vi "Save Timestamps to TXT.vi"(10 "Path To Exp":path, 11 "Timestamps (ms)":u64[](array[numeric])) -> (2 "Path To Exp out":path)   [LabVIEW 2020]
uses:
  <vilib>/Utility/file.llb/Write Delimited Spreadsheet (I64).vi
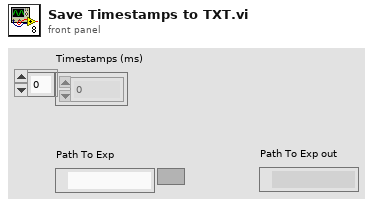
[diagram p1: front panel]
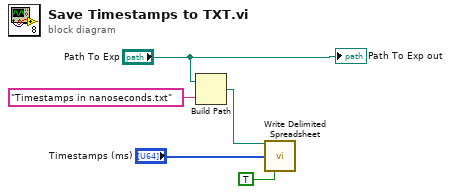
[diagram p0: block diagram]
diagram:
  n1 = Build Path(base path="Path To Exp", name or relative path="Timestamps in nanoseconds.txt") -> (appended path=w3:path)
  n2 = call-poly <vilib>:"Write Delimited Spreadsheet.vi"("file path (dialog if empty)"=w3, "1D data"="Timestamps (ms)", "transpose? (no:F)"=TRUE) -> ()  [unwired: 11 in, 2 out]
  "Path To Exp out" <- "Path To Exp"
